vi "shiftingfrequencyTest.vi"() -> ()   [LabVIEW 2012]
uses:
  <vilib>/express/express analysis/Spectral/Block/exnSpectralBlock spectral measurements RMS poly.vi
  <vilib>/express/express analysis/Spectral/Block/exnSpectralBlock spectral measurements RMS DDT.vi
  <vilib>/express/express analysis/Spectral/XNode/ExpressSpectralMeasurementsBlockNode.xnode
panel:
  out "FFT Original":waveform(dbl)(graph)
  out "Frequency Off By":dbl
  out "Output Frequency":dbl
  out "Note Frequency":dbl
  out "Note Closest To":string
  in  "Input Frequency":dbl
  out "Shifted Waveform":waveform(dbl)(graph)
  out "Original Waveform":dynamicdata(graph)
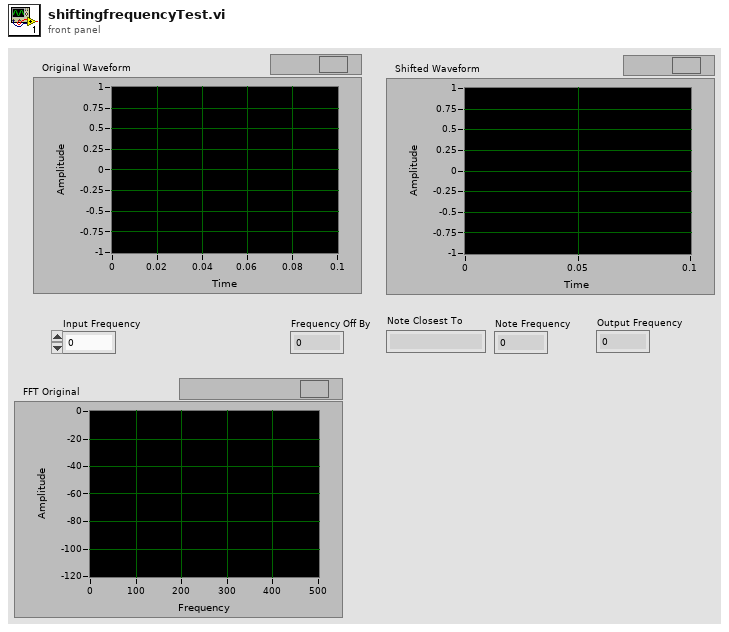
[diagram p1: front panel]
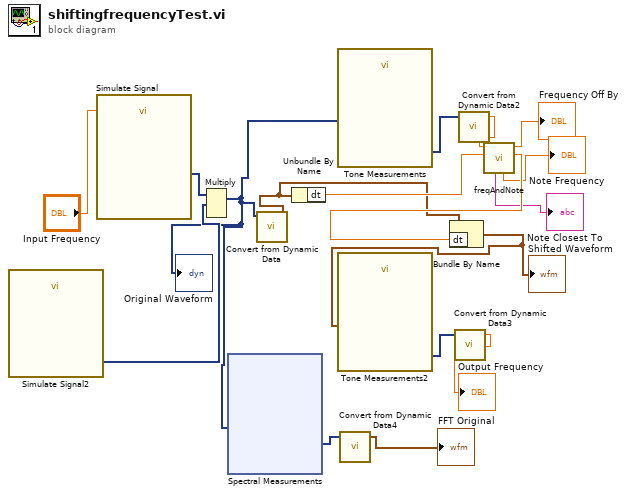
[diagram p0: block diagram]
diagram:
  n1 = call "Simulate Signal2"() -> ("Triangle"=w5:dynamicdata)  [unwired: 14 in, 1 out]
  n2 = call "Simulate Signal"("Frequency"="Input Frequency") -> ("Sine"=w4:dynamicdata)  [unwired: 13 in, 1 out]
  n3 = Multiply(1:w5, 2:w4) -> (0:w3:dynamicdata)  [unwired: 1 in, 1 out]
  "Original Waveform" <- w3
  n4 = xnode "Spectral Measurements"("Signals"=w3) -> ("FFT - (RMS)"=w2:dynamicdata)  [unwired: 1 in, 2 out]
  n5 = call "Convert from Dynamic Data"("Dynamic Data Type"=w3) -> ("Waveform"=w12:waveform(dbl))  [unwired: 3 in]
  n6 = Unbundle By Name(w12) -> ("dt"=w16:dbl)
  n7 = call "Tone Measurements"("Signals"=w3) -> ("Frequency"=w15:dynamicdata)  [unwired: 8 in, 2 out]
  n8 = call "Convert from Dynamic Data4"("Dynamic Data Type"=w2) -> ("Waveform"=→"FFT Original":waveform(dbl))  [unwired: 3 in]
  n9 = call "Convert from Dynamic Data2"("Dynamic Data Type"=w15) -> ("Scalar"=w14:dbl)  [unwired: 3 in]
  n10 = call "freqAndNote.vi"("dt Original"=w16, "Frequency In"=w14) -> ("output dt"=w13:dbl, "Frequency Off"=→"Frequency Off By":dbl, "Note Frequency"=→"Note Frequency":dbl, "Note Closest To"=→"Note Closest To":string)  [unwired: 6 in]
  n11 = Bundle By Name(cluster=w12, "dt"=w13) -> (w9:waveform(dbl))
  "Shifted Waveform" <- w9
  n12 = call "Tone Measurements2"("Signals"=w9) -> ("Frequency"=w11:dynamicdata)  [unwired: 8 in, 2 out]
  n13 = call "Convert from Dynamic Data3"("Dynamic Data Type"=w11) -> ("Scalar"=→"Output Frequency":dbl)  [unwired: 3 in]
